vi "epoll_wait.vi"(8 "error in (no error)":errorcluster, 9 "timeout ms (-1)":i32=-1, 10 "max events":u32, 11 "epfd in":i32) -> (0 "error out":errorcluster, 1 "timed out":bool, 2 "events":T1[](array[typedef]), 3 "epfd out":i32, 5 "number of ready fds":i32)   [LabVIEW 2013, in "Linux RT IPC.C.lvlib"]
uses:
  Linux RT IPC.C.lvlib
  Controls/epoll event struct.ctl
  Controls/functions.ctl
  <vilib>/NI/NI Linux RT Errno/Linux Errno.lvlib
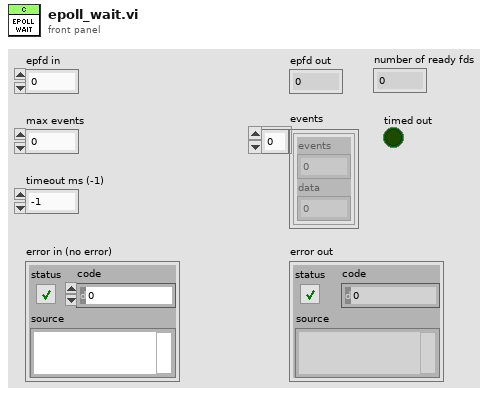
[diagram p1: front panel]
types:
  T1 = typedef "Linux RT IPC.C.lvlib/epoll event struct.ctl" = cluster{"events":u32, "data":u64}
  T2 = typedef "Linux RT IPC.C.lvlib/functions.ctl" = enum16{"unspecified", "close", "epoll_create", "epoll_ctl", "epoll_wait", "fstat", "ftruncate", "mkfifo", "mmap", "munmap", "open", "read", "shm_open", "shm_unlink", "timerfd_create", "timerfd_settime", "timerfd_gettime", "write", "unlink"}
  T3 = typedef "Linux Errno.lvlib/errno.ctl" = enum16{"NO ERROR", "EPERM", "ENOENT", "ESRCH", "EINTR", "EIO", "ENXIO", "E2BIG", "ENOEXEC", "EBADF", "ECHILD", "EAGAIN", "ENOMEM", "EACCES", "EFAULT", "ENOTBLK", "EBUSY", "EEXIST", "EXDEV", "ENODEV", "ENOTDIR", "EISDIR", "EINVAL", "ENFILE", "EMFILE", "ENOTTY", "ETXTBSY", "EFBIG", "ENOSPC", "ESPIPE", "EROFS", "EMLINK", "EPIPE", "EDOM", "ERANGE", "EDADLK", "ENAMETOOLONG", "ENOLCK", "ENOSYS", "ENOTEMPTY", "ELOOP", "EWOULDBLOCK", "ENOMSG", "EIDRM", "ECHRNG", "EL2NSYNC", "EL3HLT", "EL3RST", "ELNRNG", "EUNATCH", "ENOCSI", "EL2HLT", "EBADE", "EBADR", "EXFULL", "ENOANO", "EBADRQC", "EBADSLT", "EDEADLOCK", "EBFONT", "ENOSTR", "ENODATA", "ETIME", "ENOSR", "ENONET", "ENOPKG", "EREMOTE", "ENOLINK", "EADV", "ESRMNT", "ECOMM", "EPROTO", "EMULTIHOP", "EDOTDOT", "EBADMSG", "EOVERFLOW", "ENOTUNIQ", "EBADFD", "EREMCHG", "ELIBACC", "ELIBBAD", "ELIBSCN", "ELIBMAX", "ELIBEXEC", "ELISEQ", "ERESTART", "ESTRPIPE", "EUSERS", "ENOTSOCK", "EDESTADDRREQ", "EMSGSIZE", "EPROTOTYPE", "ENOPROTOOPT", "EPROTONOSUPPORT", "ESOCKTNOSUPPORT", "EOPNOTSUPP", "EPFNOSUPPORT", "EAFNOSUPPORT", "EADDRINUSE", "EADDRNOTAVAIL", "ENETDOWN", "ENETUNREACH", "ENETRESET", "ECONNABORTED", "ECONNRESET", "ENOBUFS", "EISCONN", "ENOTCONN", "ESHUTDOWN", "ETOOMANYREFS", "ETIMEDOUT", "ECONNREFUSED", "EHOSTDOWN", "EHOSTUNREACH", "EALREADY", "EINPROGRESS", "ESTALE", "EUCLEAN", "ENOTNAM", "ENAVAIL", "EISNAM", "EREMOTEIO", "EDQUOT", "ENOMEDIUM", "EMEDIUMTYPE", "ECANCELED", "ENOKEY", "EKEYEXPIRED", "EKEYREVOKED", "EKEYREJECTED", "EOWNERDEAD", "ENOTRECOVERABLE", "ERFKILL", "EHWPOISON", "UNDEFINED"}
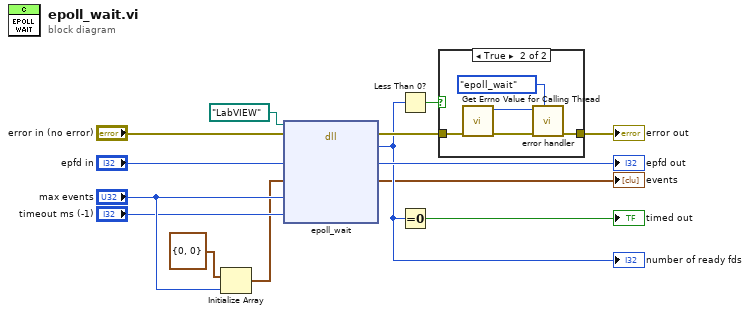
[diagram p0: block diagram]
diagram:
  n1 = Initialize Array(T1 {"events"=0, "data"=0} ("event"), "max events") -> (w2:T1[])
  n2 = dll-call lib="LabVIEW" fn="epoll_wait"(path in=path "LabVIEW", error in="error in (no error)", "epfd"="epfd in", "event"=w2, "max_events"="max events", "timeout"="timeout ms (-1)") -> (error out=w13:errorcluster, "return"=w5:i32, "epfd"=→"epfd out":i32, "event"=→"events":T1[])  [unwired: 3 in, 1 out]
  "number of ready fds" <- w5
  n3 = Less Than 0?(x=w5) -> (x < 0?=w11:bool)
  n4 = Equal To 0?(x=w5) -> (x = 0?=→"timed out":bool)
  n5 = case shown="True" w11 {
    tunnel: w13 -> [w15 w20]
    tunnel: [w15 w19] -> w12
    frame False {
    }
    frame True {
      n6 = call <vilib>:"Get Errno Value for Calling Thread.vi"("error in (no error)"=w20) -> ("error out"=w18:errorcluster, "errno"=w17:T3)  [unwired: 9 in]
      n7 = call "error handler.vi"("function (unspecified)"=functions."epoll_wait" ("function"), "error in (no error)"=w18, "errno"=w17) -> ("error out"=w19:errorcluster)  [unwired: 8 in]
    }
  }
  "error out" <- w12
